vi "Excel_Insert_Picture.vi"(6 "name":string, 7 "Shapes":refnum<k7>, 8 "error in (no error)":errorcluster, 9 "position":cluster{"Left":i32, "Top":i32}, 10 "Filename":string, 11 "Worksheet":refnum<k7>) -> (0 "error out":errorcluster)   [LabVIEW 2010, in "NI_ReportGenerationToolkit.lvlib"]
uses:
  <vilib>/addons/_office/NI_ReportGenerationToolkit.lvlib
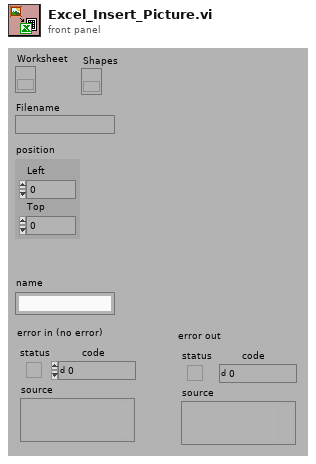
[diagram p1: front panel]
types:
  T1 = typedef "imagedata.ctl" = cluster{"image type":i32, "image depth":i32, "image":u8[], "mask":u8[], "colors":u32[], "Rectangle":cluster{"left":i16, "top":i16, "right":i16, "bottom":i16}}
  T2 = cluster{"left":i16, "top":i16, "right":i16, "bottom":i16}
  T3 = cluster{"left":dbl, "top":dbl, "right":dbl, "bottom":dbl}
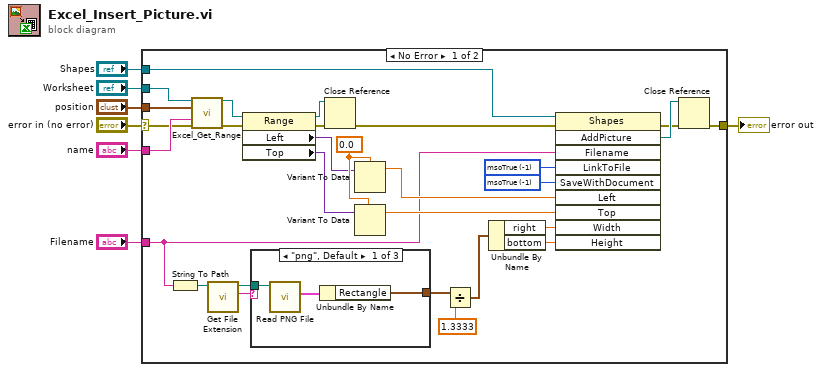
[diagram p0: block diagram]
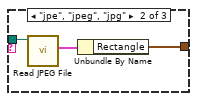
[diagram p2: hidden frame]
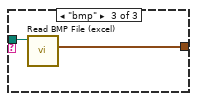
[diagram p3: hidden frame]
diagram:
  n1 = case shown="No Error" "error in (no error)" {
    selector: "error in (no error)" -> [w13 w45]
    tunnel: [w34 w45] -> w7
    tunnel: "Filename" -> [w25 _]
    tunnel: "Worksheet" -> [w16 _]
    tunnel: "name" -> [w15 _]
    tunnel: "position" -> [w14 _]
    tunnel: "Shapes" -> [w11 _]
    frame No Error {
      w30 = sgl 0.0 ("Left")
      w35 = -1 items=["msoTrue"=-1, "msoFalse"=0, "msoCTrue"=1, "msoTriStateToggle"=-3, "msoTriStateMixed"=-2] ("LinkToFile")
      w36 = -1 items=["msoTrue"=-1, "msoFalse"=0, "msoCTrue"=1, "msoTriStateToggle"=-3, "msoTriStateMixed"=-2] ("SaveWithDocument")
      n2 = String To Path(string=w25) -> (path=w10:path)
      n3 = call <vilib>:"Excel_Get_Range.vi"("Excel._Worksheet"=w16, "start"=w14, "name"=w15, "error in (no error)"=w13) -> ("Range"=w12:refnum<k7>, "error out"=w17:errorcluster)  [unwired: 1 in, 9 out]
      n4 = call <vilib>:"Get File Extension.vi"("file"=w10) -> ("lowercase file extension"=w8:string, "dup file"=w9:path)  [unwired: 1 in, 8 out]
      n5 = property class="Range"(reference=w12, error in=w17) -> (reference out=w31:refnum<k7>, error out=w32:errorcluster, "Left"=w29:variant, "Top"=w28:variant)
      n6 = case shown="\"png\", Default" w8 {
        tunnel: w9 -> [w39 w42 w44]
        tunnel: [w37 w40 w43] -> w24
        frame "png", Default {
          n7 = call <vilib>:"Read PNG File.vi"("path to PNG file"=w39) -> ("image data"=w38:T1)  [unwired: 1 in, 9 out]
          n8 = Unbundle By Name(w38) -> ("Rectangle"=w37:T2)
        }
        frame "jpe", "jpeg", "jpg" {
          n9 = call <vilib>:"Read JPEG File.vi"("path to JPEG file"=w42) -> ("image data"=w41:T1)  [unwired: 1 in, 9 out]
          n10 = Unbundle By Name(w41) -> ("Rectangle"=w40:T2)
        }
        frame "bmp" {
          n11 = call <vilib>:"Read BMP File (excel).vi"("path to BMP file"=w44) -> ("rect"=w43:T2)  [unwired: 1 in, 9 out]
        }
      }
      n12 = Close Reference(reference=w31, error in (no error)=w32) -> (error out=w19:errorcluster)
      n13 = Variant To Data(Variant=w29, type=w30) -> (data=w27:sgl)  [unwired: 1 in, 1 out]
      n14 = Variant To Data(Variant=w28, type=w30) -> (data=w26:sgl)  [unwired: 1 in, 1 out]
      n15 = Divide(x=w24, y=1.3333) -> (x/y=w22:T3)
      n16 = Unbundle By Name(w22) -> ("right"=w20:dbl, "bottom"=w21:dbl)
      n17 = invoke class="Shapes" method="AddPicture"(reference=w11, error in=w19, "Filename"=w25, "LinkToFile"=w35, "SaveWithDocument"=w36, "Left"=w27, "Top"=w26, "Width"=w20, "Height"=w21) -> (error out=w18:errorcluster, "AddPicture"=w33:refnum<k7>)  [unwired: 1 in, 8 out]
      n18 = Close Reference(reference=w33, error in (no error)=w18) -> (error out=w34:errorcluster)
    }
    frame Error {
    }
  }
  "error out" <- w7
